vi "Get AD.vi"(0 "reference in":refnum<class "AD.lvclass">, 1 "Count":i32, 5 "error in (no error)":errorcluster) -> (14 "reference out":refnum<class "AD.lvclass">, 15 "Value":dbl, 19 "error out":errorcluster)   [LabVIEW 2013, in "AD.lvclass"]
uses:
  AD.lvclass
  <vilib>/Analysis/baseanly.llb/Mean (DBL).vi
  <vilib>/Analysis/NI_AALBase.lvlib
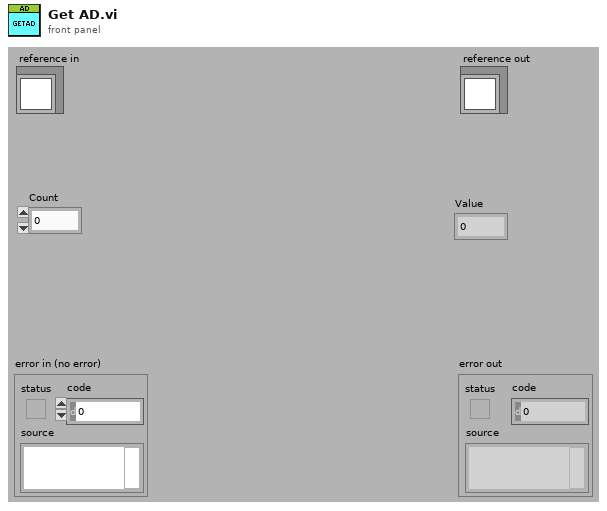
[diagram p1: front panel]
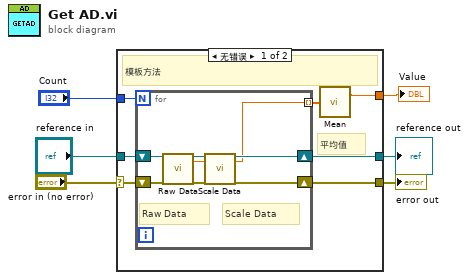
[diagram p0: block diagram]
diagram:
  n1 = case shown="无错误" "error in (no error)" {
    selector: "error in (no error)" -> [w12 w23]
    tunnel: [w7 w23] -> w5
    tunnel: [w8 w22] -> w3
    tunnel: "reference in" -> [w13 w22]
    tunnel: [w10 _] -> w2
    tunnel: "Count" -> [w9 _]
    frame No Error {
      # "平均值"
      # "模板方法"
      n2 = for {
        N: w9 -> [_]
        shift-right: [w16] -> w8
        shift-left: w13 -> [w21]
        shift-right: [w15] -> w7
        shift-left: w12 -> [w18]
        tunnel: [w14] -> w11 mode=indexing
        # "Scale Data"
        # "Raw Data"
        n3 = call-dynamic "Raw Data.vi"("reference in"=w21, "error in (no error)"=w18) -> ("reference out"=w20:refnum<class "AD.lvclass">, "Raw Data"=w19:dbl, "error out"=w17:errorcluster)  [unwired: 15 in]
        n4 = call-dynamic "Scale Data.vi"("reference in"=w20, "Raw Data"=w19, "error in (no error)"=w17) -> ("reference out"=w16:refnum<class "AD.lvclass">, "Scaled Data"=w14:dbl, "error out"=w15:errorcluster)  [unwired: 14 in]
      }
      n5 = call-poly <vilib>:"Mean.vi"("X"=w11) -> ("mean"=w10:dbl)  [unwired: 1 out]
    }
    frame Error {
    }
  }
  "error out" <- w5
  "reference out" <- w3
  "Value" <- w2
